vi "sv_Compute Shift and Low Pass Filter with IC.vi"(0 "input signal":dbl[](array[numeric]), 1 "t0":dbl, 2 "new dt":dbl, 3 "center":dbl, 4 "interpolation factor":i32, 5 "error in (no error)":errorcluster, 6 "reset? (F)":bool, 7 "delay":i32, 8 "filters":T2[](array[typedef]) {"coefficients" format="%.2f"}, 9 "initial conditions":T1, 10 "CIC settings":cluster{"Numeric":i32, i32, i32}) -> (11 "final conditions":T1, 14 "enveloped signal":dbl[](array[numeric]), 15 "t0 out":dbl, 19 "error out":errorcluster)   [LabVIEW 2017, in "SoundVib_FaultAnalysis.lvlib"]
uses:
  <vilib>/addons/Sound and Vibration/Order Analysis/Fault Analysis/SoundVib_FaultAnalysis.lvlib
  <vilib>/addons/_NISVFA/_Shared subVIs/Controls/OAT Decimation Filter.ctl
  <vilib>/addons/Sound and Vibration/Order Analysis/Adv Resampling/OAT Single Stage Decimation with IC.vi
  <vilib>/addons/Sound and Vibration/Order Analysis/Resample Order Tracking/SubVIs/OAT CIC Decimation.vi
  <vilib>/addons/Sound and Vibration/Order Analysis/Resample Order Tracking/SubVIs/oa_Interpolate Zeros Between Samples.vi
  <vilib>/addons/Sound and Vibration/Order Analysis/Resample Order Tracking/SoundVib_Resampling.lvlib
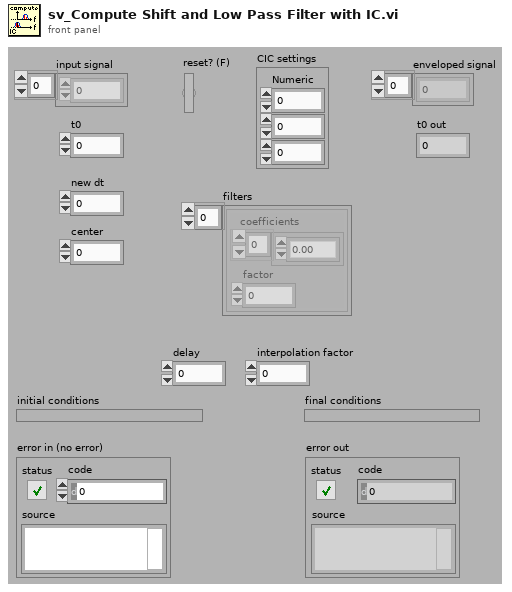
[diagram p1: front panel]
types:
  T1 = cluster{"t0":dbl, "phase":dbl, "real filter state":cluster{cluster{dbl[]}, cluster{dbl[]}[]}, "imaginary filter state":cluster{cluster{dbl[]}, cluster{dbl[]}[]}, "delay":i32}
  T2 = typedef "OAT Decimation Filter.ctl" = cluster{"coefficients":dbl[], "factor":i32}
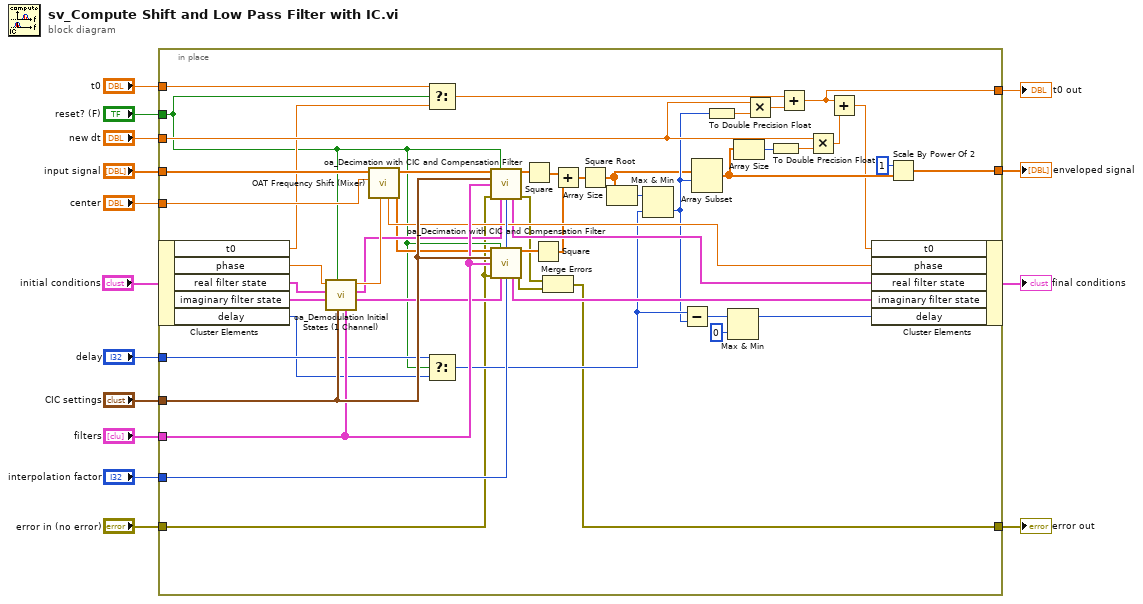
[diagram p0: block diagram]
diagram:
  n1 = in-place {
    in-place-border: "input signal" -> [w64]
    in-place-border: "center" -> [w63]
    in-place-border: "t0" -> [w62]
    in-place-border: [w61] -> w12
    in-place-border: "new dt" -> [w60]
    in-place-border: [w57] -> w10
    in-place-border: "reset? (F)" -> [w21]
    in-place-border: "CIC settings" -> [w56]
    in-place-border: "filters" -> [w55]
    in-place-border: "delay" -> [w54]
    in-place-border: "interpolation factor" -> [w53]
    in-place-border: "error in (no error)" -> [w19]
    in-place-border: [w16] -> w1
    n2 = in-place-cluster #1("initial conditions") -> ("t0"=w52:dbl, "phase"=w51:dbl, "real filter state"=w50:cluster{cluster{dbl[]}, cluster{dbl[]}[]}, "imaginary filter state"=w49:cluster{cluster{dbl[]}, cluster{dbl[]}[]}, "delay"=w48:i32)
    n3 = call <vilib>:"oa_Demodulation Initial States (1 Channel).vi"("filters"=w55, "CIC filter settings"=w56, "reset? (F)"=w21, "imaginary state in"=w49, "real state in"=w50, "phase in"=w51) -> ("imaginary state out"=w38:cluster{cluster{dbl[]}, cluster{dbl[]}[]}, "real state out"=w39:cluster{cluster{dbl[]}, cluster{dbl[]}[]}, "phase out"=w42:dbl)  [unwired: 3 in]
    n4 = call <vilib>:"OAT Frequency Shift (Mixer).vi"("initial phase"=w42, "fc"=w63, "X"=w64) -> ("imaginary"=w34:dbl[], "real"=w32:dbl[], "final phase"=w46:dbl)  [unwired: 6 in]
    n5 = Select(t=w62, s=w21, f=w52) -> (s? t:f=w31:dbl)
    n6 = Select(t=w54, s=w21, f=w48) -> (s? t:f=w37:i32)
    n7 = call <vilib>:"oa_Decimation with CIC and Compensation Filter.vi"("x[n]"=w32, "reset? (True)"=w21, "CIC decimation setting"=w56, "decimation filters"=w55, "error in (no error)"=w19, "statein"=w39, "interpolation factor"=w53) -> ("x[n] out"=w28:dbl[], "state out"=w45:cluster{cluster{dbl[]}, cluster{dbl[]}[]}, "error out"=w18:errorcluster)  [unwired: 6 in]
    n8 = call <vilib>:"oa_Decimation with CIC and Compensation Filter.vi"("x[n]"=w34, "reset? (True)"=w21, "CIC decimation setting"=w56, "decimation filters"=w55, "error in (no error)"=w19, "statein"=w38, "interpolation factor"=w53) -> ("x[n] out"=w27:dbl[], "state out"=w44:cluster{cluster{dbl[]}, cluster{dbl[]}[]}, "error out"=w17:errorcluster)  [unwired: 6 in]
    n9 = Square(x=w28) -> (x^2=w30:dbl[])
    n10 = Square(x=w27) -> (x^2=w26:dbl[])
    n11 = Merge Errors(w18, w17) -> (w16:errorcluster)
    n12 = Add(x=w30, y=w26) -> (x+y=w29:dbl[])
    n13 = Square Root(x=w29) -> (sqrt(x)=w20:dbl[])
    n14 = Array Size(array=w20) -> (size(s)=w33:i32)
    n15 = Max & Min(x=w33, y=w37) -> (min(x,y)=w23:i32)  [unwired: 1 out]
    n16 = Subtract(x=w37, y=w23) -> (x-y=w41:i32)
    n17 = Array Subset(array=w20, index=w23) -> (w58:dbl[])  [unwired: 1 in]
    n18 = To Double Precision Float(number=w23) -> (double precision float=w22:dbl)
    n19 = Max & Min(x=w41, y=0) -> (max(x,y)=w43:i32)  [unwired: 1 out]
    n20 = Array Size(array=w58) -> (size(s)=w25:i32)
    n21 = Multiply(x=w60, y=w22) -> (x*y=w36:dbl)
    n22 = To Double Precision Float(number=w25) -> (double precision float=w24:dbl)
    n23 = Add(x=w31, y=w36) -> (x+y=w61:dbl)
    n24 = Multiply(x=w60, y=w24) -> (x*y=w35:dbl)
    n25 = Add(x=w61, y=w35) -> (x+y=w47:dbl)
    n26 = in-place-cluster #1("t0"=w47, "phase"=w46, "real filter state"=w45, "imaginary filter state"=w44, "delay"=w43) -> (→"final conditions":T1)
    n27 = Scale By Power Of 2(n=1, x=w58) -> (x*2^n=w57:dbl[])
  }
  "enveloped signal" <- w10
  "t0 out" <- w12
  "error out" <- w1
